vi "Make baby.vi"(9 "Accepted?":bool, 10 "Direction":T1, 11 "Data Value Reference in":T2) -> (3 "Awesome! out":refnum<class "Awesome!.lvclass">)   [LabVIEW 2020, in "Awesome!.lvclass"]
uses:
  Awesome!.lvclass
  Common/Location Data.ctl
  Common/Common.lvlib
  Common/Map DVR.ctl
  Type Defs/Direction Enum.ctl
  Type Defs/SB Type Defs.lvlib
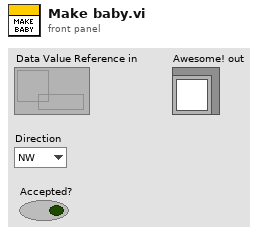
[diagram p1: front panel]
types:
  T1 = typedef "SB Type Defs.lvlib/Direction Enum.ctl" = enum16{"NW", "N", "NE", "E", "SE", "S", "SW", "W"}
  T2 = typedef "Common.lvlib/Map DVR.ctl" = refnum<data-value>
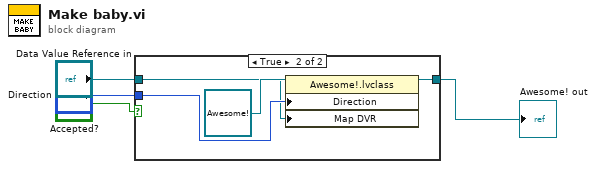
[diagram p0: block diagram]
diagram:
  n1 = case shown="True" "Accepted?" {
    tunnel: "Direction" -> [_ w8]
    tunnel: [_ w6] -> w2
    tunnel: "Data Value Reference in" -> [_ w5]
    frame False {
    }
    frame True {
      n2 = property class="Awesome!.lvclass"(reference=refnum<class "Awesome!.lvclass"> refnum ("Awesome!.lvclass"), "Direction"=w8, "Map DVR"=w5) -> (reference out=w6:refnum<class "Awesome!.lvclass">)  [unwired: 1 in, 1 out]
    }
  }
  "Awesome! out" <- w2
